vi "Ungueltiger Messwert Stoerung.vi"() -> (1 "Störung Messgerät":bool)   [LabVIEW 2020, in "AK-Schnittstelle.lvlib"]
uses:
  AK-Schnittstelle.lvlib
  Stoerungen/FGV Stoermeldungen Aktion.ctl
  Stoerungen/Stoerungen.lvlib
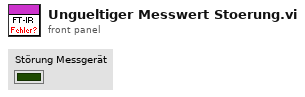
[diagram p1: front panel]
types:
  T1 = typedef "Stoerungen.lvlib/FGV Stoermeldungen Aktion.ctl" = enum16{"Initialisieren", "kommend", "gehend", "lesen", "Queue leeren", "Queue freigeben", "in Datei loggen", "Änderung zurücksetzen"}
  T2 = typedef "Stoerungen.lvlib/Stoermeldung.ctl" = cluster{"Zeitstempel":timestamp, "Nummer":i32, "Kommend":bool}
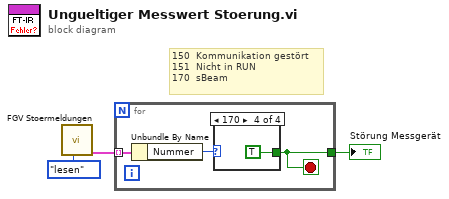
[diagram p0: block diagram]
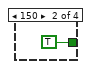
[diagram p3: hidden frame]
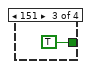
[diagram p4: hidden frame]
diagram:
  # "150  Kommunikation gestört\n151  Nicht in RUN\n170  sBeam"
  n1 = call "FGV Stoermeldungen.vi"("Aktion"=FGV_Stoermeldungen_Aktion."lesen") -> ("Anzeige Array"=w2:T2[])  [unwired: 7 in, 3 out]
  n2 = for {
    tunnel: w2 -> [w6] mode=indexing
    tunnel: [w4] -> w1
    stop <- w4 stop-if-true
    n3 = Unbundle By Name(w6) -> ("Nummer"=w5:i32)
    n4 = case shown="170" w5 {
      tunnel: [_ TRUE TRUE TRUE] -> w4
      frame 0, Default {
      }
      frame 150 {
      }
      frame 151 {
      }
      frame 170 {
      }
    }
  }
  "Störung Messgerät" <- w1
